vi "Main FPGA 8-axis with Limits.vi"() -> ()   [LabVIEW 2013]
uses:
  <vilib>/Motion/MotorControl/_s/nism.interpretControlRegister.stateTransition.ctl
  <vilib>/Platform/TimedLoop/XDataNode/timing_clust.ctl
  <vilib>/Platform/TimedLoop/XDataNode/nitl_modes.ctl
  <vilib>/Platform/TimedLoop/XDataNode/wakeup.ctl
  <vilib>/Motion/MotorControl/_s/nism.digitalInputs.portA.ctl
  <vilib>/rvi/Emulation/niFpgaSctlEmulationGetInTimedLoop.vi
  <vilib>/rvi/Emulation/niFpgaEmulationReportErrorSimple.vi
  <vilib>/rvi/Emulation/niFpgaGetClockAttributes.vi
  <vilib>/rvi/Emulation/niFpgaCriticalErrorInLSC.vi
  Global FPGA.vi
  <vilib>/rvi/eio/common/nirviEmuTemplateMethod_errors.vi
  <vilib>/Motion/SoftMotion/Synchronization/nism.rioScan.generateSyncScan.vi
  <vilib>/rvi/Emulation/niFpgaProcessEmulError.vi
  <vilib>/Motion/MotorControl/_s/nism.interpretControlRegister.indexed.vi
  <vilib>/Motion/MotorControl/_s/nism.generateStatusRegister.indexed.vi
  <vilib>/Motion/MotorControl/_s/nism.mdo.read.positionLoopSyncData.vi
  <vilib>/Motion/MotorControl/_s/nism.mdo.read.splineData.vi
  <vilib>/Motion/MotorControl/_s/nism.splineInterpolation.fxp.3.index.vi
  <vilib>/Motion/MotorControl/_s/nism.mdo.handler.indexed.vi
  <vilib>/Motion/MotorControl/_s/nism.digitalFilter.u8.vi
  <vilib>/Motion/MotorControl/_s/nism.interpretDIOControl.portA.single.2.vi
  <vilib>/Motion/MotorControl/_s/nism.generateDIOStatus.portA.single.vi
  <vilib>/Platform/TimedLoop/XDataNode/XDataNode.xnode
  <vilib>/eio/EIONode/EIONode.xnode
  <vilib>/Motion/MotorControl/NI_SoftMotion_MotorControlIP.lvlib
  <vilib>/Platform/TimedLoop/XDataNode/XDNodeRunTimeDep.lvlib
  <vilib>/Motion/SoftMotion/Synchronization/NI_SoftMotion_Synchronization.lvlib
panel:
  in  "Axis Digital Inputs (U8)":u8[](array[numeric])=[0, 0, 0, 0, 0, 0, 0, 0]
  out "Axis Positions":fxp<+/-,64,32>[](array[numeric])
  in  "STEP or CW? (T=STEP)":bool
  out "Drive Enable":bool[](array[boolean])
  in  "Enable Watchdog":bool
  in  "Pet Watchdog":bool
  in  "Watchdog Timeout Period (ticks)":u64=40000000 format="%.0p"
  out "Watchdog Timed Out?":bool
  out "Time Since Last Pet":u64
  in  "Enable value":bool
  in  "Drive Enable override?":bool
  out "State":T1=enum."Start --> Initializing" caption="state transition"
  in  "Sync Value":bool
  in  "Sync Enable override?":bool
  in  "Invert direction?":bool
  out "Sync is Fault":bool
  out "Sync is Locked":bool
  in  "minimum pulse":u16=40
  # "Synchronization Loop"
  # "Control Status Loop"
  # "Notes: \n1. This VI provides the communication interface between the NI SoftMotion Engine and the LabVIEW FPGA Module. You must compile this VI for a specific FPGA target before use. After compiling, run the VI before running any of the Express VI examples. For information on moving this example to another FPGA target, refer to ni.com/info and enter info code fpgaex.\n\n2. Only use the Reset Axis button if you are unable to communicate with the axis by any other means. This button resets the device state machine and other VIs to a known state. After resetting the axis, switch the NI Scan Engine from Active Mode to Configuration Mode, then back to Active Mode, before attempting to enable the axis."
  # "(These two buttons \nare for testing\npurposes.)"
  # "(These two buttons \nare for testing\npurposes.)"
  # "Step/Direction Loop"
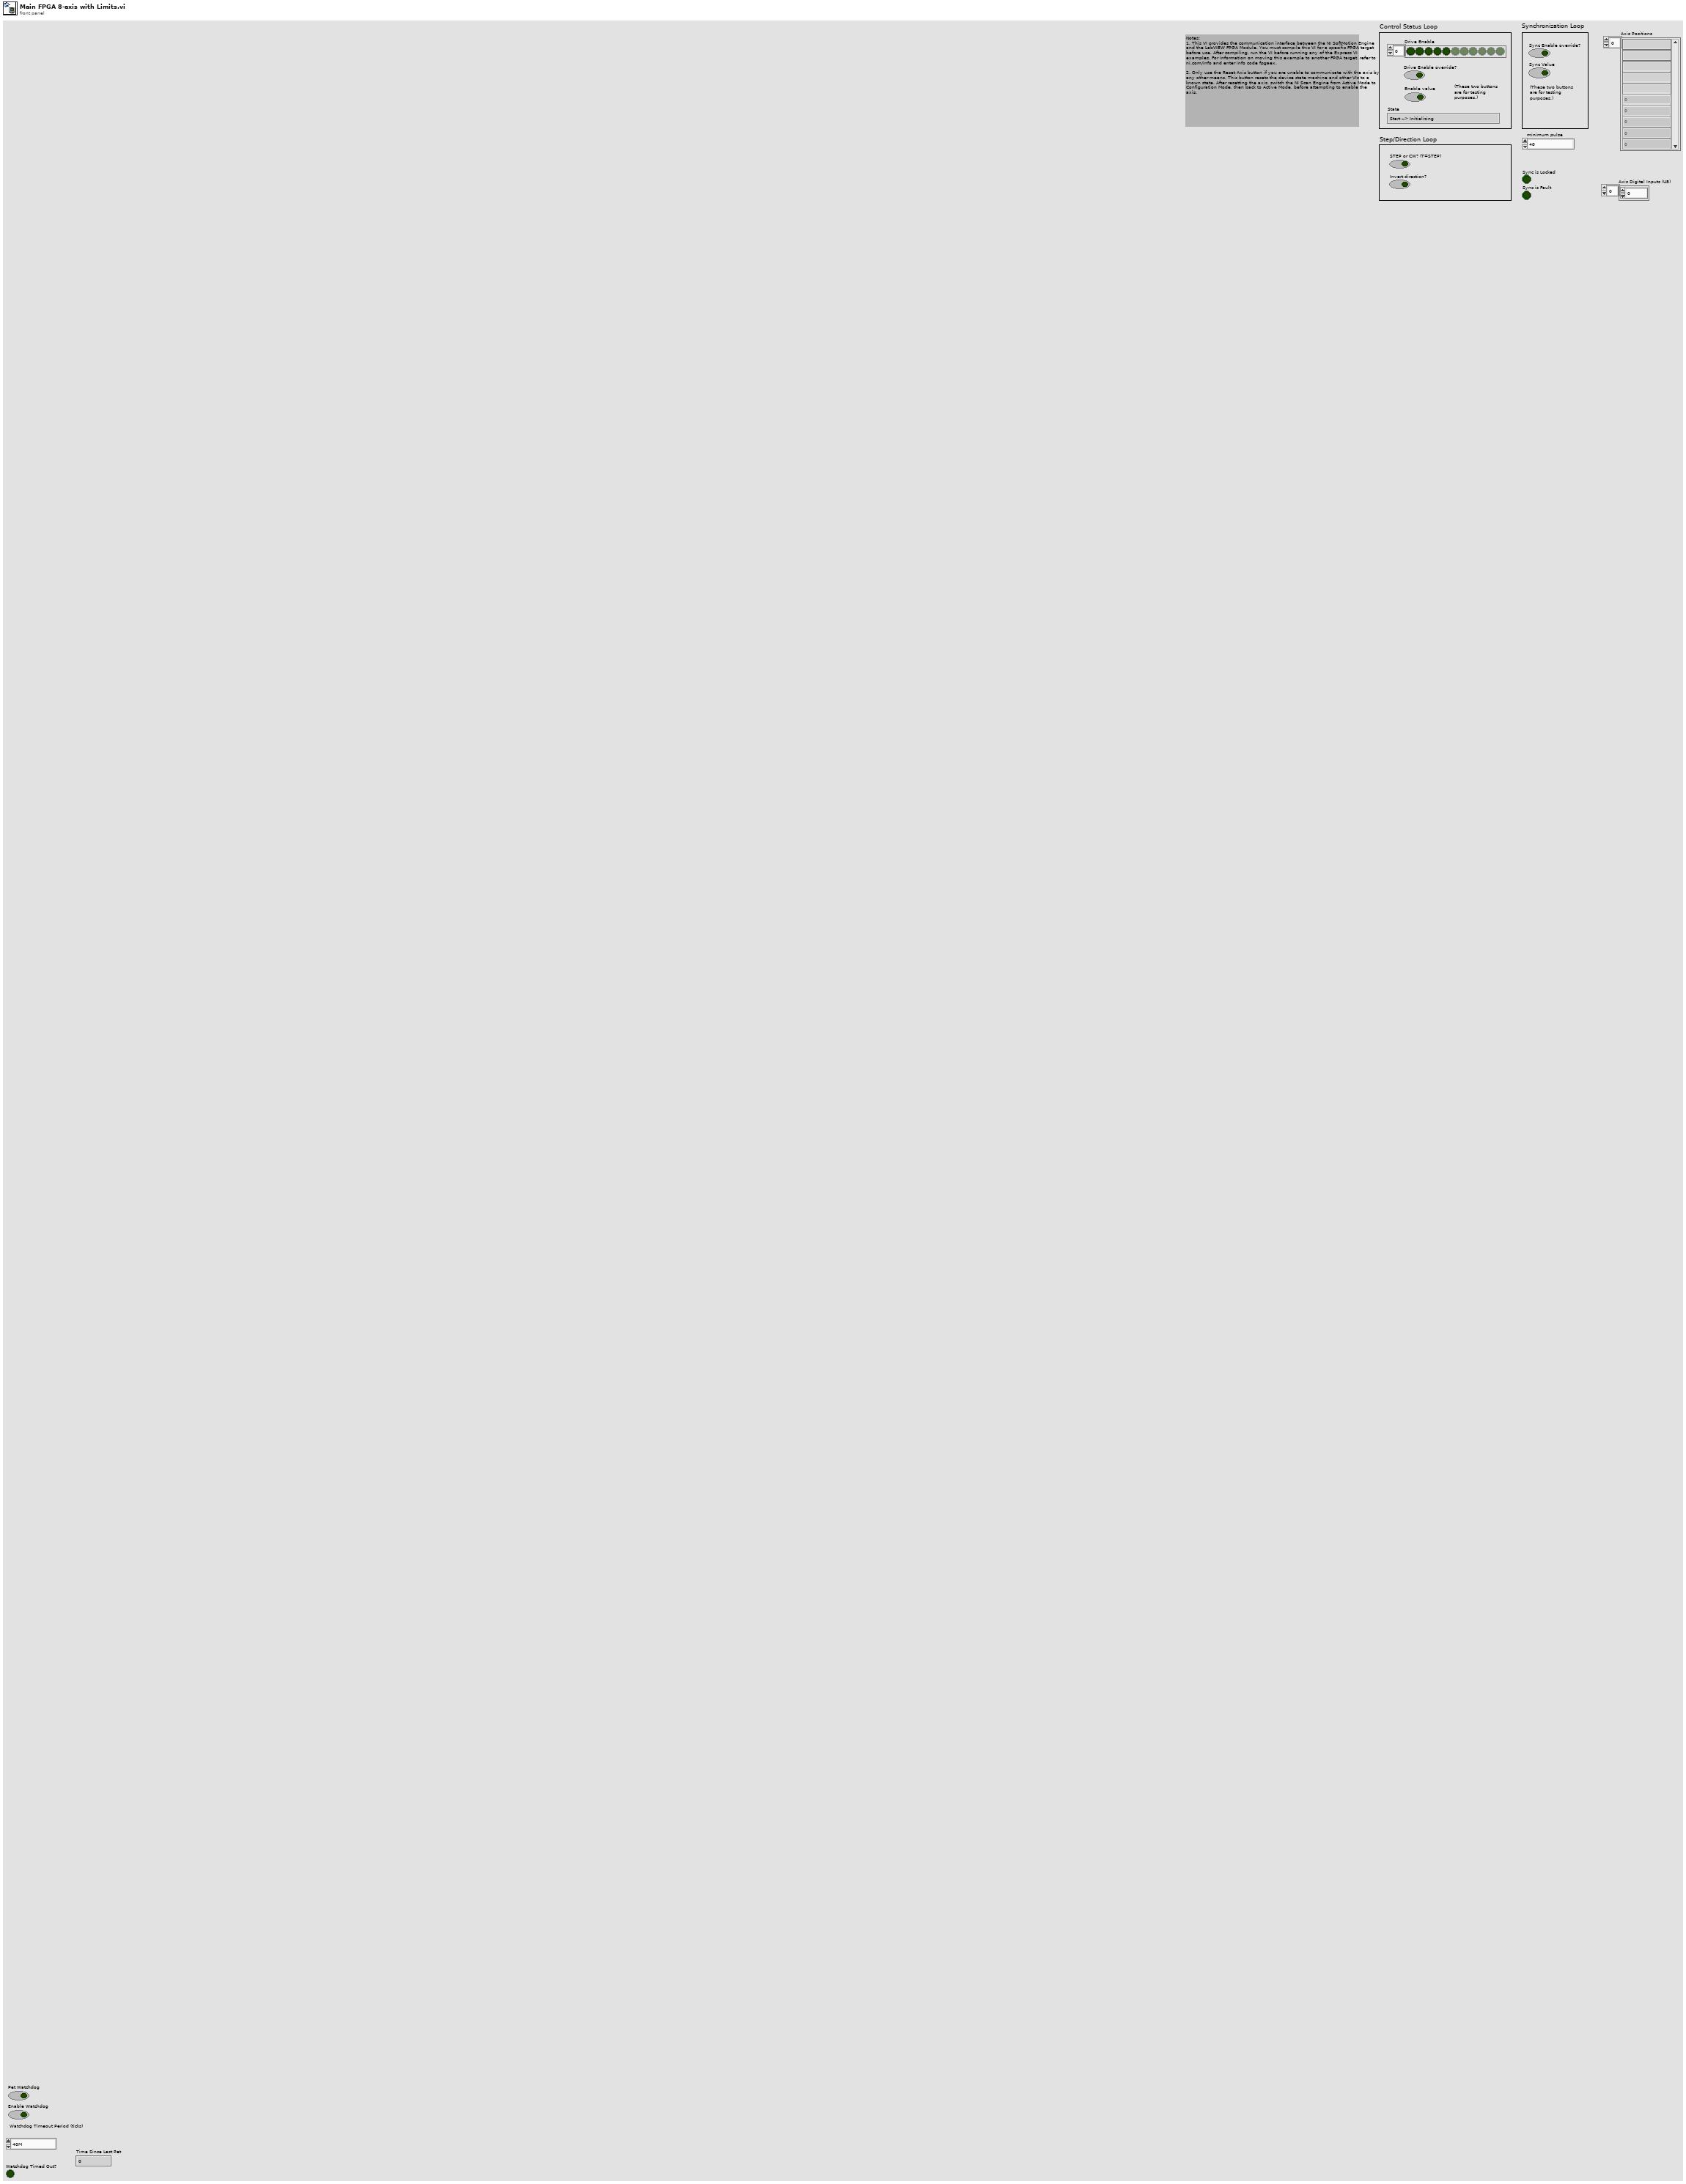
[diagram p1: front panel]
types:
  T1 = typedef "NI_SoftMotion_MotorControlIP.lvlib/nism.interpretControlRegister.stateTransition.ctl" = enum8{"Invalid", "Start --> Initializing", "Initializing --> Disabled", "Disabled --> Ready To Switch On", "Ready To Switch On --> Switched On", "Ready To Switch On --> Disable", "Switched On --> Operation Enable", "Switched On --> Ready To Switch On", "Switched On --> Disabled", "Operation Enable --> Switched On", "Operation Enable --> Ready To Switch On", "Operation Enable --> Disabled", "Fault --> Disabled", "Any --> Fault", "None"}
  T2 = typedef "NI_SoftMotion_MotorControlIP.lvlib/nism.mdo.splineData.ctl" = cluster{"spline type":T3, "traj per/spline per":u16, "spline per/traj per":fxp<+,32,0>}
  T3 = typedef "nism.splineInterpolation.type.ctl" = u16
  T4 = typedef "NI_SoftMotion_Synchronization.lvlib/nism.softmotionScan.timerConfig.ctl" = cluster{"Target Period (clocks)":u16, "Host Period / Target Period":u16}
  T5 = typedef "NI_SoftMotion_Synchronization.lvlib/nism.softmotionScan.timerControl.ctl" = cluster{"SM Scan":bool, "SM Scan Count":u32, "SM Scan Enabled":bool}
  T6 = typedef "XDNodeRunTimeDep.lvlib/timing_clust.ctl" = cluster{"Expected End [f-1]":u64, "Actual End [f-1]":u64, "Finished Late? [f-1]":bool, "Expected End [i-1]":u64, "Actual End [i-1]":u64, "Finished Late? [i-1]":bool, "Expected Start [i]":u64, "Actual Start [i]":u64, "Expected Start [f]":u64, "Actual Start [f]":u64, "Source Name":string, "Structure Name":string, "Period":i64, "Deadline":i64, "Offset":i64, "Start":i64, "Priority":i32, "Timeout":i32, "Mode":T7, "Wakeup Reason":T8, "Error":errorcluster, "Source Type":string, "Secondary Source Type":string, "Global End Time":u64, "Global Start Time":u64, "Frame Duration":u64, "Iteration Duration":u64, "Assigned CPU":i32, "I/O Scan Engine Mode":u32}
  T7 = typedef "XDNodeRunTimeDep.lvlib/nitl_modes.ctl" = enum32{"No Change", "Process missed periods, maintain original phase", "Discard missed periods, maintain original phase", "Process missed periods, ignore original phase", "Discard missed periods, ignore original phase"}
  T8 = typedef "XDNodeRunTimeDep.lvlib/wakeup.ctl" = enum32{"Normal", "Aborted", "Asynchronous wakeup", "Timing source error", "Timed loop error", "Timeout"}
  T9 = typedef "NI_SoftMotion_MotorControlIP.lvlib/nism.digitalInputs.portA.ctl" = cluster{"reverse limit":bool, "forward limit":bool, "home switch":bool, "digital input 0":bool, "digital input 1":bool, "digital input 2":bool, "digital input 3":bool}
  T10 = typedef "NI_SoftMotion_MotorControlIP.lvlib/nism.dio.portA.config.2.ctl" = cluster{"digital filter (us)":u16[], "safe state":enum16{"Low", "High", "No Change"}[]}
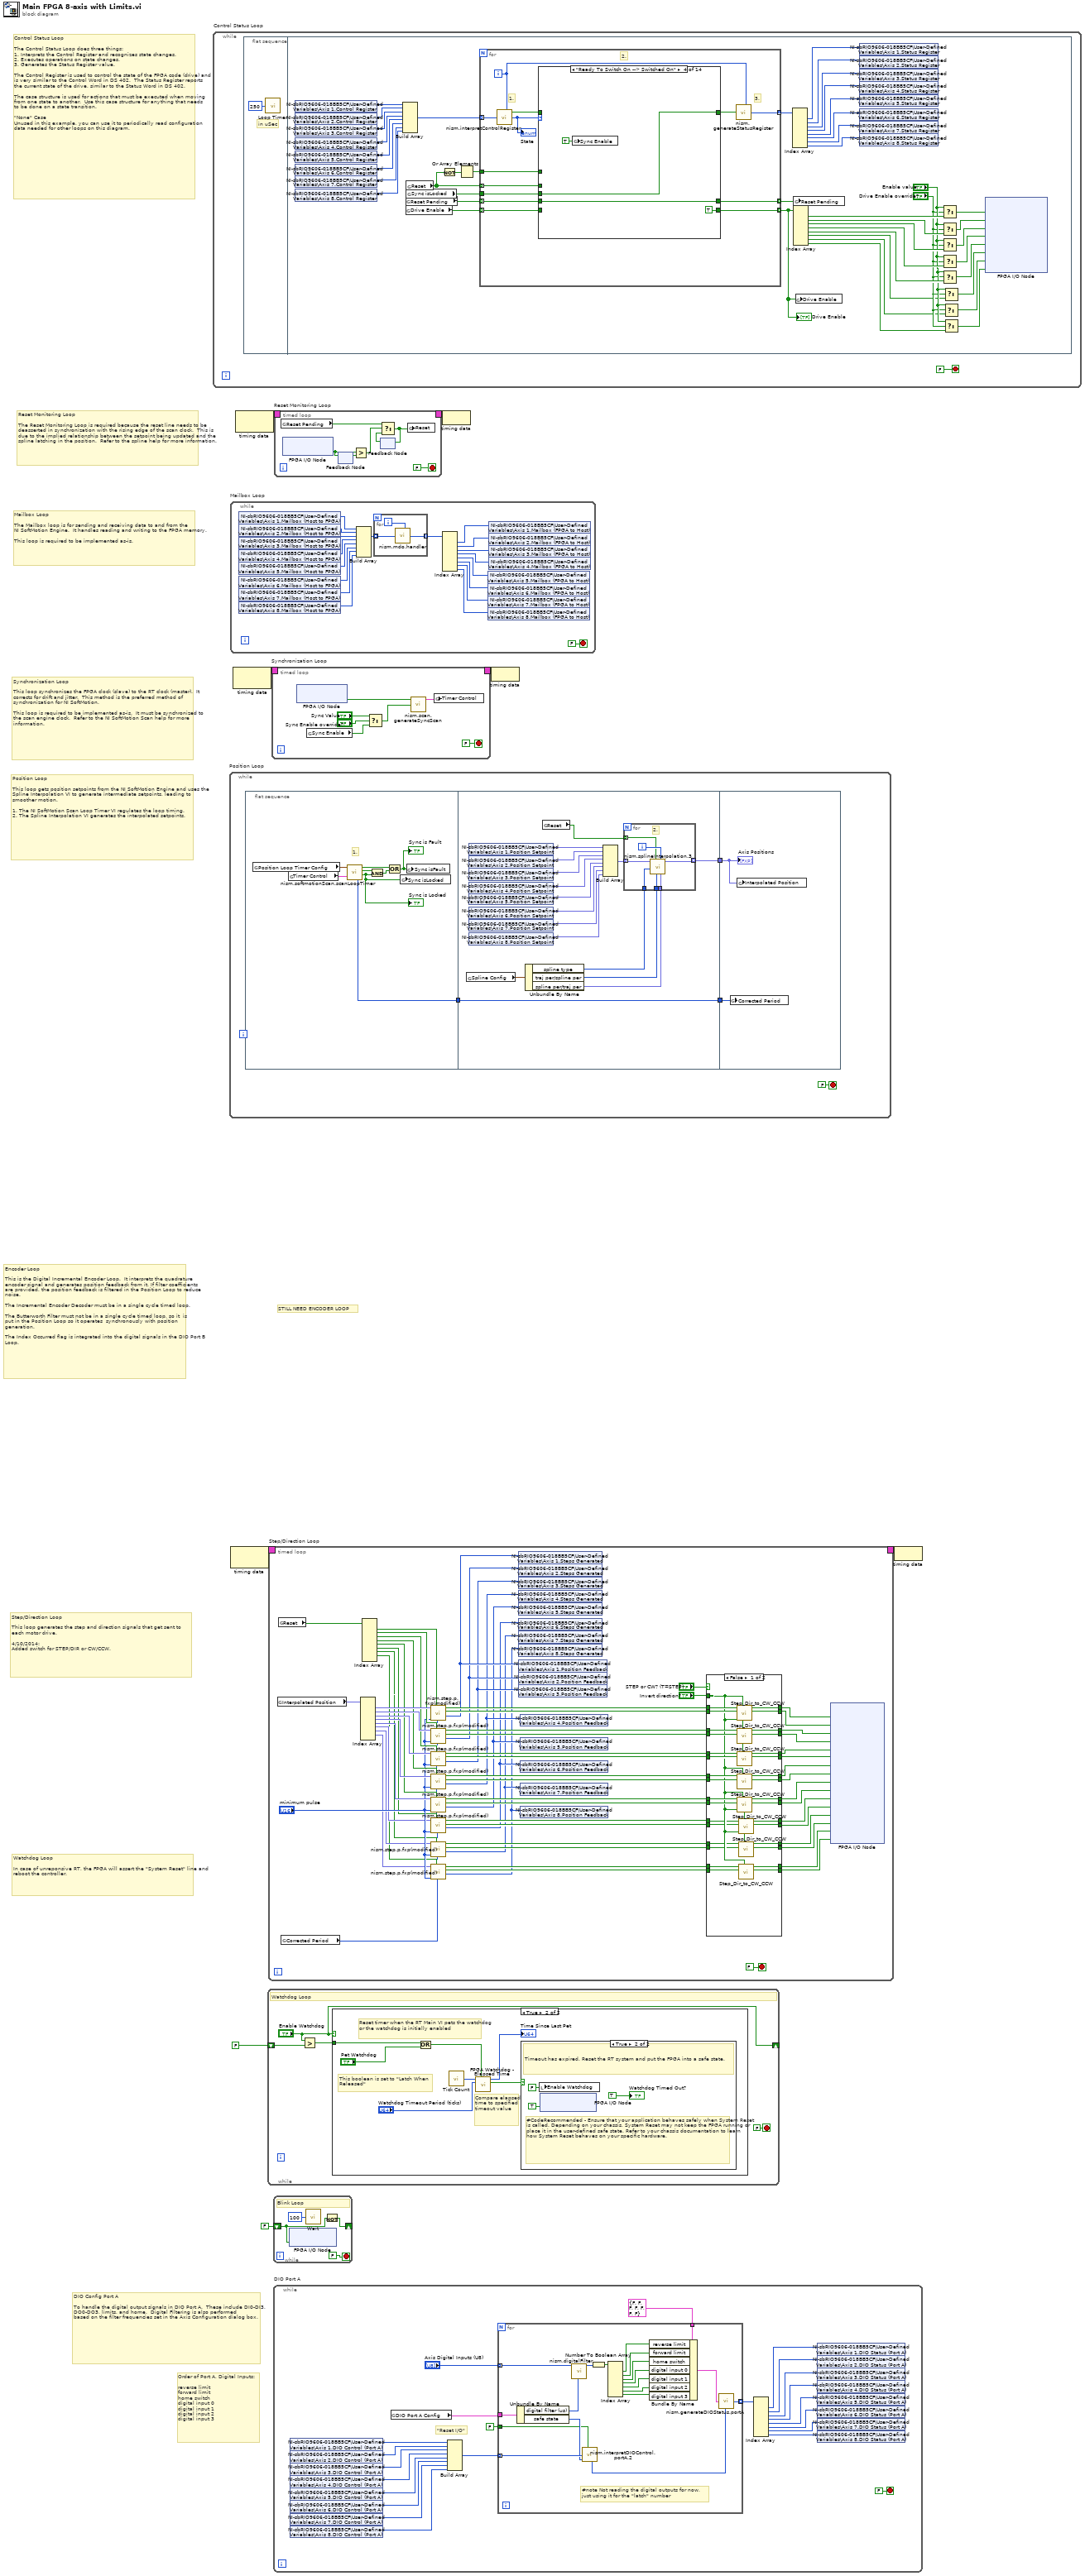
[diagram p0: block diagram]
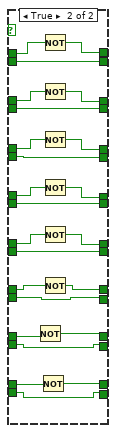
[diagram p5: hidden frame]
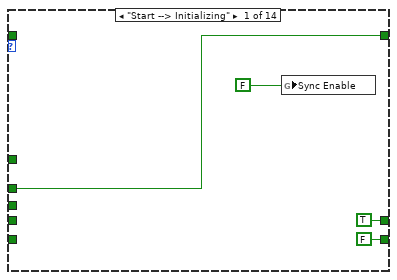
[diagram p6: hidden frame]
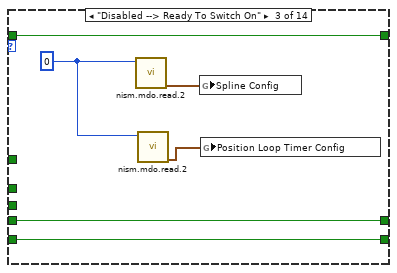
[diagram p8: hidden frame]
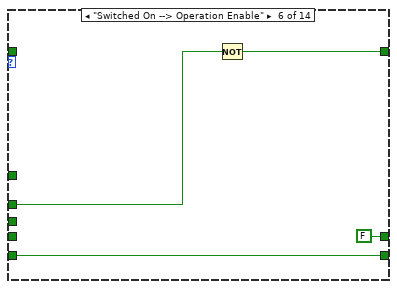
[diagram p10: hidden frame]
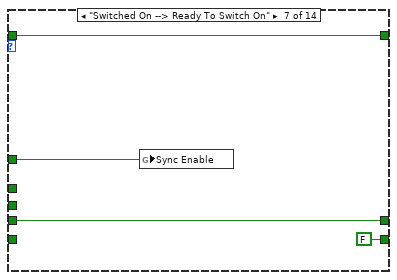
[diagram p11: hidden frame]
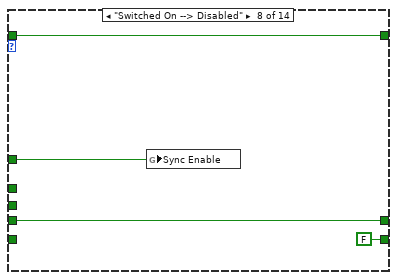
[diagram p12: hidden frame]
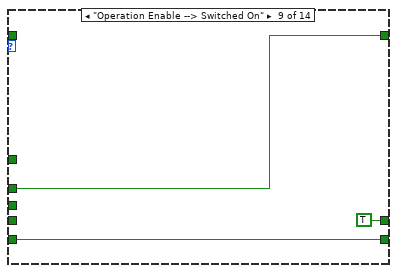
[diagram p13: hidden frame]
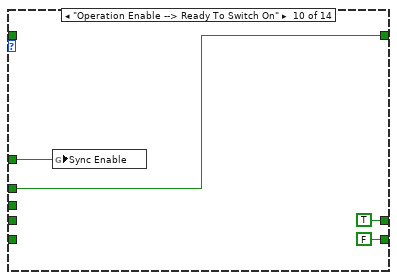
[diagram p14: hidden frame]
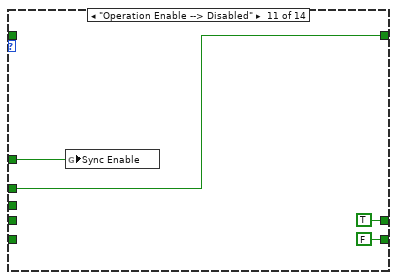
[diagram p15: hidden frame]
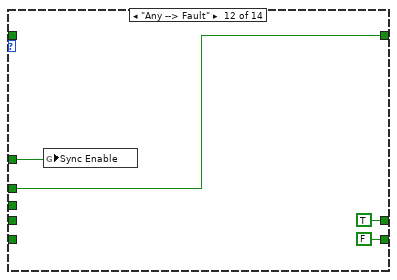
[diagram p16: hidden frame]
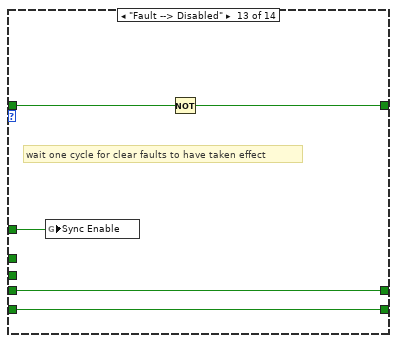
[diagram p17: hidden frame]
diagram:
  # "STILL NEED ENCODER LOOP"
  # "DIO Config Port A\n\nTo handle the digital output signals in DIO Port A.  These include DI0-DI3, DO0-DO3, limits, and home.  Digital Filtering is also performed\nbased on the filter frequencies set in the Axis Configuration dialog box."
  # "Order of Port A, Digital Inputs:\n\nreverse limit\nforward limit\nhome switch\ndigital input 0\ndigital input 1\ndigital input 2\ndigital input 3"
  # "Encoder Loop\n\nThis is the Digital Incremental Encoder Loop.  It interprets the quadrature encoder signal and generates position feedback from it. If filter coefficients are provided, the position feedback is filtered in the Position Loop to reduce noise.\n\nThe Incremental Encoder Decoder must be in a single cycle timed loop.\n\nThe Butterworth Filter must not be in a single cycle timed loop, so it  is\nput in the Position Loop so it operates  synchronously with position generation.\n\nThe Index Occurred flag is integrated into the digital signals in the DIO Port B Loop."
  # "Watchdog Loop\n\nIn case of unreponsive RT, the FPGA will assert the \"System Reset\" line and reboot the controller."
  # "Step/Direction Loop\n\nThis loop generates the step and direction signals that get sent to \neach motor drive.\n\n4/10/2014:\nAdded switch for STEP/DIR or CW/CCW."
  # "Position Loop\n\nThis loop gets position setpoints from the NI SoftMotion Engine and uses the Spline Interpolation VI to generate intermediate setpoints, leading to smoother motion.\n\n1. The NI SoftMotion Scan Loop Timer VI regulates the loop timing. \n2. The Spline Interpolation VI generates the interpolated setpoints."
  # "Synchronization Loop\n\nThis loop synchronizes the FPGA clock (slave) to the RT clock (master).  It corrects for drift and jitter.  This method is the preferred method of synchronization for NI SoftMotion.\n\nThis loop is required to be implemented as-is.  It must be synchronized to the scan engine clock.  Refer to the NI SoftMotion Scan help for more information."
  # "Mailbox Loop\n\nThe Mailbox loop is for sending and receiving data to and from the \nNI SoftMotion Engine.  It handles reading and writing to the FPGA memory.\n\nThis loop is required to be implemented as-is."
  # "Reset Monitoring Loop\n\nThe Reset Monitoring Loop is required because the reset line needs to be deasserted in synchronization with the rising edge of the scan clock.  This is due to the implied relationship between the setpoint being updated and the spline latching in the position.  Refer to the spline help for more information."
  # "Control Status Loop\n\nThe Control Status Loop does three things:\n1. Interprets the Control Register and recognizes state changes.\n2. Executes operations on state changes.\n3. Generates the Status Register value.\n\nThe Control Register is used to control the state of the FPGA code (drive) and is very similar to the Control Word in DS 402.  The Status Register reports the current state of the drive, similar to the Status Word in DS 402.\n\nThe case structure is used for actions that must be executed when moving from one state to another.  Use this case structure for anything that needs to be done on a state transition.\n\n\"None\" Case\nUnused in this example, you can use it to periodically read configuration data needed for other loops on this diagram."
  n1 = while "Control Status Loop" {
    stop <- FALSE stop-if-true
    n2 = flat-sequence {
      frame #0 {
        # "in uSec"
        n3 = call "Loop Timer"("Count(uSec)"=u32 250) -> ()  [unwired: 1 out]
      }
      frame #1 {
        n4 = shared-variable "NI-sbRIO9606-018BB5CF\\User-Defined Variables\\Axis 1.Control Register"() -> (w44:u32)  [unwired: 1 in, 1 out]
        n5 = shared-variable "NI-sbRIO9606-018BB5CF\\User-Defined Variables\\Axis 2.Control Register"() -> (w43:u32)  [unwired: 1 in, 1 out]
        n6 = shared-variable "NI-sbRIO9606-018BB5CF\\User-Defined Variables\\Axis 3.Control Register"() -> (w42:u32)  [unwired: 1 in, 1 out]
        n7 = shared-variable "NI-sbRIO9606-018BB5CF\\User-Defined Variables\\Axis 4.Control Register"() -> (w41:u32)  [unwired: 1 in, 1 out]
        n8 = shared-variable "NI-sbRIO9606-018BB5CF\\User-Defined Variables\\Axis 5.Control Register"() -> (w40:u32)  [unwired: 1 in, 1 out]
        n9 = shared-variable "NI-sbRIO9606-018BB5CF\\User-Defined Variables\\Axis 6.Control Register"() -> (w24:u32)  [unwired: 1 in, 1 out]
        n10 = shared-variable "NI-sbRIO9606-018BB5CF\\User-Defined Variables\\Axis 7.Control Register"() -> (w23:u32)  [unwired: 1 in, 1 out]
        n11 = shared-variable "NI-sbRIO9606-018BB5CF\\User-Defined Variables\\Axis 8.Control Register"() -> (w22:u32)  [unwired: 1 in, 1 out]
        n12 = Build Array(w44, w43, w42, w41, w40, w24, w23, w22) -> (w53:u32[])
        n13 = global read "Global FPGA.vi" "Reset Pending"() -> (w48:bool[])
        n14 = global read "Global FPGA.vi" "Drive Enable"() -> (w47:bool[])
        n15 = global read "Global FPGA.vi" "Reset"() -> (w49:bool[])
        n16 = global read "Global FPGA.vi" "Sync isLocked"() -> (w54:bool)
        n17 = Not(x=w49) -> (.not. x?=w51:bool[])
        n18 = Or Array Elements(Boolean array=w51) -> (logical OR=w50:bool)
        n19 = for {
          tunnel: w49 -> [w62] mode=indexing
          tunnel: w54 -> [w61]
          tunnel: w53 -> [w63] mode=indexing
          tunnel: [w60] -> w45 mode=indexing
          tunnel: [w59] -> w52 mode=indexing
          tunnel: [w58] -> w46 mode=indexing
          tunnel: w50 -> [w57]
          tunnel: w48 -> [w56] mode=indexing
          tunnel: w47 -> [w55] mode=indexing
          i -> [w64]
          # "3."
          # "2."
          # "1."
          n20 = call-poly <vilib>:"nism.interpretControlRegister.vi"("control register"=w63, "axis index"=w64) -> ("transition occurred"=w65:bool, "state transition"=w66:T1)  [unwired: 6 in]
          "State" <- w66
          n21 = case shown="\"Ready To Switch On --> Switched On\"" w66 {
            tunnel: w65 -> [_ w74 w80 _ w87 _ w95 w99 _ _ _ _ w119 _]
            tunnel: [w71 w74 w80 w82 w87 w91 w95 w99 w101 w104 w108 w112 w118 _] -> w67
            tunnel: w62 -> [w71 _ _ _ _ w90 _ _ w101 w104 w108 w112 _ _]
            tunnel: w61 -> [_ _ _ w82 _ _ _ _ _ _ _ _ _ _]
            tunnel: [TRUE ("Write.Reset Pending") w73 w76 w81 w86 FALSE ("Write.Reset Pending") w92 w96 TRUE ("Write.Reset Pending") TRUE ("Write.Reset Pending") TRUE ("Write.Reset Pending") TRUE ("Write.Reset Pending") w116 w121] -> w59
            tunnel: [FALSE ("Write.Drive Enable") w72 w75 TRUE ("Write.Drive Enable") w85 w88 FALSE ("Write.Drive Enable") FALSE ("Write.Drive Enable") w100 FALSE ("Write.Drive Enable") FALSE ("Write.Drive Enable") FALSE ("Write.Drive Enable") w115 w120] -> w58
            tunnel: w57 -> [_ _ _ _ _ _ w93 w97 _ w103 w107 w111 w117 _]
            tunnel: w56 -> [_ w73 w76 w81 w86 _ w92 w96 _ _ _ _ w116 w121]
            tunnel: w55 -> [_ w72 w75 _ w85 w88 _ _ w100 _ _ _ w115 w120]
            frame "Start --> Initializing" {
              n22 = global write "Global FPGA.vi" "Sync Enable"(FALSE ("Sync Enable")) -> ()
            }
            frame "Initializing --> Disabled" {
            }
            frame "Disabled --> Ready To Switch On" {
              w78 = 0 ("axis index")
              n23 = call-poly <vilib>:"nism.mdo.read.2.vi"("axis index"=w78) -> ("spline"=w79:T2)  [unwired: 10 in]
              n24 = call-poly <vilib>:"nism.mdo.read.2.vi"("axis index"=w78) -> ("position loop sync"=w77:T4)  [unwired: 10 in]
              n25 = global write "Global FPGA.vi" "Spline Config"(w79) -> ()
              n26 = global write "Global FPGA.vi" "Position Loop Timer Config"(w77) -> ()
            }
            frame "Ready To Switch On --> Switched On" {
              n27 = global write "Global FPGA.vi" "Sync Enable"(TRUE ("Sync Enable")) -> ()
            }
            frame "Ready To Switch On --> Disable" {
            }
            frame "Switched On --> Operation Enable" {
              n28 = Not(x=w90) -> (.not. x?=w91:bool)
            }
            frame "Switched On --> Ready To Switch On" {
              n29 = global write "Global FPGA.vi" "Sync Enable"(w93) -> ()
            }
            frame "Switched On --> Disabled" {
              n30 = global write "Global FPGA.vi" "Sync Enable"(w97) -> ()
            }
            frame "Operation Enable --> Switched On" {
            }
            frame "Operation Enable --> Ready To Switch On" {
              n31 = global write "Global FPGA.vi" "Sync Enable"(w103) -> ()
            }
            frame "Operation Enable --> Disabled" {
              n32 = global write "Global FPGA.vi" "Sync Enable"(w107) -> ()
            }
            frame "Any --> Fault" {
              n33 = global write "Global FPGA.vi" "Sync Enable"(w111) -> ()
            }
            frame "Fault --> Disabled" {
              # "wait one cycle for clear faults to have taken effect"
              n34 = global write "Global FPGA.vi" "Sync Enable"(w117) -> ()
              n35 = Not(x=w119) -> (.not. x?=w118:bool)
            }
            frame "None", Default {
            }
          }
          n36 = call-poly <vilib>:"nism.generateStatusRegister.vi"("transition success"=w67, "axis index"=w64) -> ("status register"=w60:u32)  [unwired: 7 in]
        }
        "Drive Enable" <- w46
        n37 = Index Array(array=w45) -> (element #1=w39:u32, element #2=w38:u32, element #3=w37:u32, element #4=w36:u32, element #5=w35:u32, element #6=w21:u32, element #7=w20:u32, element #8=w19:u32)  [unwired: 8 in]
        n38 = global write "Global FPGA.vi" "Reset Pending"(w52) -> ()
        n39 = Index Array(array=w46) -> (element #1=w34:bool, element #2=w32:bool, element #3=w30:bool, element #4=w28:bool, element #5=w26:bool, element #6=w16:bool, element #7=w15:bool, element #8=w14:bool)  [unwired: 8 in]
        n40 = global write "Global FPGA.vi" "Drive Enable"(w46) -> ()
        n41 = shared-variable "NI-sbRIO9606-018BB5CF\\User-Defined Variables\\Axis 1.Status Register"(w39) -> ()  [unwired: 1 in, 1 out]
        n42 = shared-variable "NI-sbRIO9606-018BB5CF\\User-Defined Variables\\Axis 2.Status Register"(w38) -> ()  [unwired: 1 in, 1 out]
        n43 = shared-variable "NI-sbRIO9606-018BB5CF\\User-Defined Variables\\Axis 3.Status Register"(w37) -> ()  [unwired: 1 in, 1 out]
        n44 = shared-variable "NI-sbRIO9606-018BB5CF\\User-Defined Variables\\Axis 4.Status Register"(w36) -> ()  [unwired: 1 in, 1 out]
        n45 = shared-variable "NI-sbRIO9606-018BB5CF\\User-Defined Variables\\Axis 5.Status Register"(w35) -> ()  [unwired: 1 in, 1 out]
        n46 = shared-variable "NI-sbRIO9606-018BB5CF\\User-Defined Variables\\Axis 6.Status Register"(w21) -> ()  [unwired: 1 in, 1 out]
        n47 = shared-variable "NI-sbRIO9606-018BB5CF\\User-Defined Variables\\Axis 7.Status Register"(w20) -> ()  [unwired: 1 in, 1 out]
        n48 = shared-variable "NI-sbRIO9606-018BB5CF\\User-Defined Variables\\Axis 8.Status Register"(w19) -> ()  [unwired: 1 in, 1 out]
        n49 = Select(t="Enable value", s="Drive Enable override?", f=w34) -> (s? t:f=w33:bool)
        n50 = Select(t="Enable value", s="Drive Enable override?", f=w32) -> (s? t:f=w31:bool)
        n51 = Select(t="Enable value", s="Drive Enable override?", f=w30) -> (s? t:f=w29:bool)
        n52 = Select(t="Enable value", s="Drive Enable override?", f=w28) -> (s? t:f=w27:bool)
        n53 = Select(t="Enable value", s="Drive Enable override?", f=w26) -> (s? t:f=w25:bool)
        n54 = Select(t="Enable value", s="Drive Enable override?", f=w16) -> (s? t:f=w13:bool)
        n55 = Select(t="Enable value", s="Drive Enable override?", f=w15) -> (s? t:f=w12:bool)
        n56 = Select(t="Enable value", s="Drive Enable override?", f=w14) -> (s? t:f=w11:bool)
        n57 = xnode "FPGA I/O Node"("Axis1_Servo On"=w33, "Axis2_Servo On"=w31, "Axis3_Servo On"=w29, "Axis4_Servo On"=w27, "Axis5_Servo On"=w25, "RMC/DIO1"=w13, "RMC/DIO2"=w12, "RMC/DIO3"=w11) -> ()  [unwired: 8 in, 8 out]
      }
    }
  }
  n58 = while "Position Loop" {
    stop <- FALSE stop-if-true
    n59 = flat-sequence {
      tunnel: [w126] -> w122
      tunnel: [w143] -> w124
      tunnel: [w142] -> w123
      tunnel: w122 -> [w142]
      tunnel: w124 -> [w157]
      tunnel: w123 -> [w158]
      frame #0 {
        # "1."
        n60 = global read "Global FPGA.vi" "Position Loop Timer Config"() -> (w128:T4)
        n61 = global read "Global FPGA.vi" "Timer Control"() -> (w127:T5)
        n62 = call <vilib>:"nism.softmotionScan.scanLoopTimer.vi"("Timer Control"=w127, "Timer Config"=w128) -> ("Scan Running?"=w130:bool, "Finished Late?"=w132:bool, "Fault Occurred?"=w133:bool, "Corrected Period"=w126:u16)  [unwired: 5 in, 1 out]
        "Sync is Locked" <- w130
        n63 = Compound Arithmetic op=AND(w132, w130) -> (w131:bool)
        n64 = Compound Arithmetic op=OR(w133, w131) -> (w129:bool)
        "Sync is Fault" <- w129
        n65 = global write "Global FPGA.vi" "Sync isLocked"(w130) -> ()
        n66 = global write "Global FPGA.vi" "Sync isFault"(w129) -> ()
      }
      frame #1 {
        n67 = global read "Global FPGA.vi" "Spline Config"() -> (w145:T2)
        n68 = shared-variable "NI-sbRIO9606-018BB5CF\\User-Defined Variables\\Axis 1.Position Setpoint"() -> (w141:fxp<+/-,64,32>)  [unwired: 1 in, 1 out]
        n69 = shared-variable "NI-sbRIO9606-018BB5CF\\User-Defined Variables\\Axis 2.Position Setpoint"() -> (w140:fxp<+/-,64,32>)  [unwired: 1 in, 1 out]
        n70 = shared-variable "NI-sbRIO9606-018BB5CF\\User-Defined Variables\\Axis 3.Position Setpoint"() -> (w139:fxp<+/-,64,32>)  [unwired: 1 in, 1 out]
        n71 = shared-variable "NI-sbRIO9606-018BB5CF\\User-Defined Variables\\Axis 4.Position Setpoint"() -> (w138:fxp<+/-,64,32>)  [unwired: 1 in, 1 out]
        n72 = shared-variable "NI-sbRIO9606-018BB5CF\\User-Defined Variables\\Axis 5.Position Setpoint"() -> (w137:fxp<+/-,64,32>)  [unwired: 1 in, 1 out]
        n73 = shared-variable "NI-sbRIO9606-018BB5CF\\User-Defined Variables\\Axis 6.Position Setpoint"() -> (w136:fxp<+/-,64,32>)  [unwired: 1 in, 1 out]
        n74 = shared-variable "NI-sbRIO9606-018BB5CF\\User-Defined Variables\\Axis 7.Position Setpoint"() -> (w135:fxp<+/-,64,32>)  [unwired: 1 in, 1 out]
        n75 = shared-variable "NI-sbRIO9606-018BB5CF\\User-Defined Variables\\Axis 8.Position Setpoint"() -> (w134:fxp<+/-,64,32>)  [unwired: 1 in, 1 out]
        n76 = Unbundle By Name(w145) -> ("spline type"=w149:T3, "traj per/spline per"=w148:u16, "spline per/traj per"=w147:fxp<+,32,0>)
        n77 = global read "Global FPGA.vi" "Reset"() -> (w144:bool[])
        n78 = Build Array(w141, w140, w139, w138, w137, w136, w135, w134) -> (w146:fxp<+/-,64,32>[])
        n79 = for {
          tunnel: w149 -> [w156]
          tunnel: w148 -> [w155]
          tunnel: w147 -> [w154]
          tunnel: w144 -> [w151] mode=indexing
          tunnel: w146 -> [w153] mode=indexing
          tunnel: [w150] -> w143 mode=indexing
          i -> [w152]
          # "2."
          n80 = call-poly <vilib>:"nism.splineInterpolation.3.vi"("1 / calls per sample"=w154, "index"=w152, "calls per sample"=w155, "reset"=w151, "spline type"=w156, "x"=w153) -> ("xi"=w150:fxp<+/-,64,32>)  [unwired: 5 in]
        }
      }
      frame #2 {
        n81 = global write "Global FPGA.vi" "Corrected Period"(w158) -> ()
        n82 = global write "Global FPGA.vi" "Interpolated Position"(w157) -> ()
        "Axis Positions" <- w157
      }
    }
  }
  n83 = while "Mailbox Loop" {
    stop <- FALSE stop-if-true
    n84 = shared-variable "NI-sbRIO9606-018BB5CF\\User-Defined Variables\\Axis 1.Mailbox (Host to FPGA)"() -> (w174:u64)  [unwired: 1 in, 1 out]
    n85 = shared-variable "NI-sbRIO9606-018BB5CF\\User-Defined Variables\\Axis 2.Mailbox (Host to FPGA)"() -> (w173:u64)  [unwired: 1 in, 1 out]
    n86 = shared-variable "NI-sbRIO9606-018BB5CF\\User-Defined Variables\\Axis 3.Mailbox (Host to FPGA)"() -> (w172:u64)  [unwired: 1 in, 1 out]
    n87 = shared-variable "NI-sbRIO9606-018BB5CF\\User-Defined Variables\\Axis 4.Mailbox (Host to FPGA)"() -> (w171:u64)  [unwired: 1 in, 1 out]
    n88 = shared-variable "NI-sbRIO9606-018BB5CF\\User-Defined Variables\\Axis 5.Mailbox (Host to FPGA)"() -> (w170:u64)  [unwired: 1 in, 1 out]
    n89 = shared-variable "NI-sbRIO9606-018BB5CF\\User-Defined Variables\\Axis 6.Mailbox (Host to FPGA)"() -> (w164:u64)  [unwired: 1 in, 1 out]
    n90 = shared-variable "NI-sbRIO9606-018BB5CF\\User-Defined Variables\\Axis 7.Mailbox (Host to FPGA)"() -> (w163:u64)  [unwired: 1 in, 1 out]
    n91 = shared-variable "NI-sbRIO9606-018BB5CF\\User-Defined Variables\\Axis 8.Mailbox (Host to FPGA)"() -> (w162:u64)  [unwired: 1 in, 1 out]
    n92 = Build Array(w174, w173, w172, w171, w170, w164, w163, w162) -> (w176:u64[])
    n93 = for {
      tunnel: w176 -> [w180] mode=indexing
      tunnel: [w179] -> w175 mode=indexing
      i -> [w178]
      n94 = call-poly <vilib>:"nism.mdo.handler.vi"("mbox (host to fpga)"=w180, "axis index"=w178) -> ("mbox (fpga to host)"=w179:u64)  [unwired: 7 in]
    }
    n95 = Index Array(array=w175) -> (element #1=w169:u64, element #2=w168:u64, element #3=w167:u64, element #4=w166:u64, element #5=w165:u64, element #6=w161:u64, element #7=w160:u64, element #8=w159:u64)  [unwired: 8 in]
    n96 = shared-variable "NI-sbRIO9606-018BB5CF\\User-Defined Variables\\Axis 6.Mailbox (FPGA to Host)"(w161) -> ()  [unwired: 1 in, 1 out]
    n97 = shared-variable "NI-sbRIO9606-018BB5CF\\User-Defined Variables\\Axis 7.Mailbox (FPGA to Host)"(w160) -> ()  [unwired: 1 in, 1 out]
    n98 = shared-variable "NI-sbRIO9606-018BB5CF\\User-Defined Variables\\Axis 8.Mailbox (FPGA to Host)"(w159) -> ()  [unwired: 1 in, 1 out]
    n99 = shared-variable "NI-sbRIO9606-018BB5CF\\User-Defined Variables\\Axis 5.Mailbox (FPGA to Host)"(w165) -> ()  [unwired: 1 in, 1 out]
    n100 = shared-variable "NI-sbRIO9606-018BB5CF\\User-Defined Variables\\Axis 1.Mailbox (FPGA to Host)"(w169) -> ()  [unwired: 1 in, 1 out]
    n101 = shared-variable "NI-sbRIO9606-018BB5CF\\User-Defined Variables\\Axis 2.Mailbox (FPGA to Host)"(w168) -> ()  [unwired: 1 in, 1 out]
    n102 = shared-variable "NI-sbRIO9606-018BB5CF\\User-Defined Variables\\Axis 3.Mailbox (FPGA to Host)"(w167) -> ()  [unwired: 1 in, 1 out]
    n103 = shared-variable "NI-sbRIO9606-018BB5CF\\User-Defined Variables\\Axis 4.Mailbox (FPGA to Host)"(w166) -> ()  [unwired: 1 in, 1 out]
  }
  n104 = node-c288() -> (w8:T6)  [unwired: 1 in]
  n105 = node-c288() -> (w6:T6)  [unwired: 1 in]
  n106 = node-c288() -> (w4:T6)  [unwired: 1 in]
  n107 = while "RT Watchdog Loop" {
    shift-right: ["Enable Watchdog"] -> _
    shift-left: FALSE ("Enable RT Watchdog") -> [w184]
    stop <- FALSE stop-if-true
    # "Watchdog Loop"
    n108 = Greater?(x="Enable Watchdog", y=w184) -> (0:w181:bool)
    n109 = case shown="True" "Enable Watchdog" {
      tunnel: w181 -> [_ w187]
      frame False {
        # "This loop has to be explicitly enabled from the RT Main VI.  This reduces the possiblity of an endless reboot cycle."
      }
      frame True {
        # "This boolean is set to \"Latch When Released\""
        # "Compare elapsed time to specified timeout value"
        # "Reset timer when the RT Main VI pets the watchdog or the watchdog is initially enabled"
        n110 = Or(x=w187, y="Pet Watchdog") -> (x .or. y?=w186:bool)
        n111 = call "Tick Count"() -> ("Tick Count(Ticks)"=w190:u32)
        n112 = call "FPGA Watchdog - Elapsed Time.vi"("Reset"=w186, "Timeout Period"="Watchdog Timeout Period (ticks)", "Current Time"=w190) -> ("Timeout"=w185:bool, "Elapsed Time"=→"Time Since Last Pet":u64)  [unwired: 7 in]
        n113 = case shown="True" w185 {
          frame False {
            # "Timeout has not expired."
          }
          frame True {
            # "#CodeRecommended - Ensure that your application behaves safely when System Reset is called. Depending on your chassis, System Reset may not keep the FPGA running or place it in the user-defined safe state. Refer to your chassis documentation to learn how System Reset behaves on your specific hardware."
            # "Timeout has expired. Reset the RT system and put the FPGA into a safe state."
            n114 = local write "Enable Watchdog"(FALSE ("Enable RT Watchdog")) -> ()
            n115 = xnode "FPGA I/O Node"("System Reset"=TRUE ("RT Reset on Watchdog Failure?")) -> ()  [unwired: 1 in, 1 out]
            "Watchdog Timed Out?" <- TRUE ("Watchdog Timed Out?")
          }
        }
      }
    }
  }
  n116 = timed-loop "Step/Direction Loop" {
    timing: w8 -> [_]
    timing-out: [_] -> w7
    stop <- FALSE stop-if-true
    n117 = global read "Global FPGA.vi" "Interpolated Position"() -> (w256:fxp<+/-,64,32>[])
    n118 = global read "Global FPGA.vi" "Reset"() -> (w250:bool[])
    n119 = global read "Global FPGA.vi" "Corrected Period"() -> (w203:u16)
    n120 = Index Array(array=w256) -> (element #1=w255:fxp<+/-,64,32>, element #2=w254:fxp<+/-,64,32>, element #3=w253:fxp<+/-,64,32>, element #4=w252:fxp<+/-,64,32>, element #5=w251:fxp<+/-,64,32>, element #6=w215:fxp<+/-,64,32>, element #7=w214:fxp<+/-,64,32>, element #8=w213:fxp<+/-,64,32>)  [unwired: 9 in, 1 out]
    n121 = Index Array(array=w250) -> (element #1=w249:bool, element #2=w248:bool, element #3=w247:bool, element #4=w246:bool, element #5=w245:bool, element #6=w212:bool, element #7=w211:bool, element #8=w210:bool)  [unwired: 9 in, 1 out]
    n122 = call "nism.step.p.fxp(modified).vi"("calls per sample"=w203, "reset"=w249, "minimum pulse"="minimum pulse", "position setpoint"=w255) -> ("steps generated"=w202:i32, "step"=w243:bool, "direction"=w244:bool)  [unwired: 4 in, 1 out]
    n123 = call "nism.step.p.fxp(modified).vi"("calls per sample"=w203, "reset"=w248, "minimum pulse"="minimum pulse", "position setpoint"=w254) -> ("steps generated"=w201:i32, "step"=w241:bool, "direction"=w242:bool)  [unwired: 4 in, 1 out]
    n124 = call "nism.step.p.fxp(modified).vi"("calls per sample"=w203, "reset"=w247, "minimum pulse"="minimum pulse", "position setpoint"=w253) -> ("steps generated"=w200:i32, "step"=w239:bool, "direction"=w240:bool)  [unwired: 4 in, 1 out]
    n125 = call "nism.step.p.fxp(modified).vi"("calls per sample"=w203, "reset"=w246, "minimum pulse"="minimum pulse", "position setpoint"=w252) -> ("steps generated"=w199:i32, "step"=w237:bool, "direction"=w238:bool)  [unwired: 4 in, 1 out]
    n126 = call "nism.step.p.fxp(modified).vi"("calls per sample"=w203, "reset"=w245, "minimum pulse"="minimum pulse", "position setpoint"=w251) -> ("steps generated"=w198:i32, "step"=w235:bool, "direction"=w236:bool)  [unwired: 4 in, 1 out]
    n127 = call "nism.step.p.fxp(modified).vi"("calls per sample"=w203, "reset"=w212, "minimum pulse"="minimum pulse", "position setpoint"=w215) -> ("steps generated"=w197:i32, "step"=w221:bool, "direction"=w222:bool)  [unwired: 4 in, 1 out]
    n128 = call "nism.step.p.fxp(modified).vi"("calls per sample"=w203, "reset"=w211, "minimum pulse"="minimum pulse", "position setpoint"=w214) -> ("steps generated"=w196:i32, "step"=w219:bool, "direction"=w220:bool)  [unwired: 4 in, 1 out]
    n129 = call "nism.step.p.fxp(modified).vi"("calls per sample"=w203, "reset"=w210, "minimum pulse"="minimum pulse", "position setpoint"=w213) -> ("steps generated"=w195:i32, "step"=w217:bool, "direction"=w218:bool)  [unwired: 4 in, 1 out]
    n130 = shared-variable "NI-sbRIO9606-018BB5CF\\User-Defined Variables\\Axis 1.Steps Generated"(w202) -> ()  [unwired: 1 in, 1 out]
    n131 = shared-variable "NI-sbRIO9606-018BB5CF\\User-Defined Variables\\Axis 2.Steps Generated"(w201) -> ()  [unwired: 1 in, 1 out]
    n132 = shared-variable "NI-sbRIO9606-018BB5CF\\User-Defined Variables\\Axis 3.Steps Generated"(w200) -> ()  [unwired: 1 in, 1 out]
    n133 = shared-variable "NI-sbRIO9606-018BB5CF\\User-Defined Variables\\Axis 4.Steps Generated"(w199) -> ()  [unwired: 1 in, 1 out]
    n134 = shared-variable "NI-sbRIO9606-018BB5CF\\User-Defined Variables\\Axis 5.Steps Generated"(w198) -> ()  [unwired: 1 in, 1 out]
    n135 = shared-variable "NI-sbRIO9606-018BB5CF\\User-Defined Variables\\Axis 6.Steps Generated"(w197) -> ()  [unwired: 1 in, 1 out]
    n136 = shared-variable "NI-sbRIO9606-018BB5CF\\User-Defined Variables\\Axis 7.Steps Generated"(w196) -> ()  [unwired: 1 in, 1 out]
    n137 = shared-variable "NI-sbRIO9606-018BB5CF\\User-Defined Variables\\Axis 8.Steps Generated"(w195) -> ()  [unwired: 1 in, 1 out]
    n138 = shared-variable "NI-sbRIO9606-018BB5CF\\User-Defined Variables\\Axis 1.Position Feedback"(w202) -> ()  [unwired: 1 in, 1 out]
    n139 = shared-variable "NI-sbRIO9606-018BB5CF\\User-Defined Variables\\Axis 2.Position Feedback"(w201) -> ()  [unwired: 1 in, 1 out]
    n140 = shared-variable "NI-sbRIO9606-018BB5CF\\User-Defined Variables\\Axis 3.Position Feedback"(w200) -> ()  [unwired: 1 in, 1 out]
    n141 = shared-variable "NI-sbRIO9606-018BB5CF\\User-Defined Variables\\Axis 4.Position Feedback"(w199) -> ()  [unwired: 1 in, 1 out]
    n142 = shared-variable "NI-sbRIO9606-018BB5CF\\User-Defined Variables\\Axis 5.Position Feedback"(w198) -> ()  [unwired: 1 in, 1 out]
    n143 = shared-variable "NI-sbRIO9606-018BB5CF\\User-Defined Variables\\Axis 6.Position Feedback"(w197) -> ()  [unwired: 1 in, 1 out]
    n144 = shared-variable "NI-sbRIO9606-018BB5CF\\User-Defined Variables\\Axis 7.Position Feedback"(w196) -> ()  [unwired: 1 in, 1 out]
    n145 = shared-variable "NI-sbRIO9606-018BB5CF\\User-Defined Variables\\Axis 8.Position Feedback"(w195) -> ()  [unwired: 1 in, 1 out]
    n146 = case shown="False" "STEP or CW? (T=STEP)" {
      tunnel: w244 -> [w290 w322]
      tunnel: w243 -> [w289 w312]
      tunnel: w242 -> [w288 w320]
      tunnel: w241 -> [w287 w310]
      tunnel: w240 -> [w286 w318]
      tunnel: w239 -> [w285 w308]
      tunnel: w238 -> [w284 w316]
      tunnel: w237 -> [w283 w306]
      tunnel: w236 -> [w282 w314]
      tunnel: w235 -> [w281 w304]
      tunnel: "Invert direction?" -> [w270 w323]
      tunnel: [w280 w321] -> w233
      tunnel: [w279 w311] -> w224
      tunnel: [w278 w319] -> w232
      tunnel: [w277 w309] -> w231
      tunnel: [w276 w317] -> w230
      tunnel: [w275 w307] -> w229
      tunnel: [w274 w315] -> w228
      tunnel: [w273 w305] -> w227
      tunnel: [w272 w313] -> w226
      tunnel: [w271 w303] -> w225
      tunnel: w222 -> [w269 w302]
      tunnel: w221 -> [w268 w301]
      tunnel: w220 -> [w267 w300]
      tunnel: w219 -> [w266 w299]
      tunnel: w218 -> [w265 w298]
      tunnel: w217 -> [w264 w297]
      tunnel: [w263 w296] -> w209
      tunnel: [w262 w295] -> w208
      tunnel: [w260 w294] -> w207
      tunnel: [w261 w293] -> w206
      tunnel: [w259 w292] -> w205
      tunnel: [w258 w291] -> w204
      frame False {
        n147 = call "Step_Dir_to_CW_CCW.vi"("invert"=w270, "step"=w289, "direction"=w290) -> ("CCW"=w279:bool, "CW"=w280:bool)  [unwired: 7 in]
        n148 = call "Step_Dir_to_CW_CCW.vi"("invert"=w270, "step"=w287, "direction"=w288) -> ("CCW"=w277:bool, "CW"=w278:bool)  [unwired: 7 in]
        n149 = call "Step_Dir_to_CW_CCW.vi"("invert"=w270, "step"=w285, "direction"=w286) -> ("CCW"=w275:bool, "CW"=w276:bool)  [unwired: 7 in]
        n150 = call "Step_Dir_to_CW_CCW.vi"("invert"=w270, "step"=w283, "direction"=w284) -> ("CCW"=w273:bool, "CW"=w274:bool)  [unwired: 7 in]
        n151 = call "Step_Dir_to_CW_CCW.vi"("invert"=w270, "step"=w281, "direction"=w282) -> ("CCW"=w271:bool, "CW"=w272:bool)  [unwired: 7 in]
        n152 = call "Step_Dir_to_CW_CCW.vi"("invert"=w270, "step"=w268, "direction"=w269) -> ("CCW"=w262:bool, "CW"=w263:bool)  [unwired: 7 in]
        n153 = call "Step_Dir_to_CW_CCW.vi"("invert"=w270, "step"=w266, "direction"=w267) -> ("CCW"=w261:bool, "CW"=w260:bool)  [unwired: 7 in]
        n154 = call "Step_Dir_to_CW_CCW.vi"("invert"=w270, "step"=w264, "direction"=w265) -> ("CCW"=w258:bool, "CW"=w259:bool)  [unwired: 7 in]
      }
      frame True {
        n155 = case shown="False" w323 {
          tunnel: w322 -> [w339 w363]
          tunnel: [w339 w362] -> w321
          tunnel: w320 -> [w337 w361]
          tunnel: [w337 w360] -> w319
          tunnel: w318 -> [w335 w359]
          tunnel: [w335 w358] -> w317
          tunnel: w316 -> [w333 w357]
          tunnel: [w333 w356] -> w315
          tunnel: w314 -> [w331 w355]
          tunnel: [w331 w354] -> w313
          tunnel: w312 -> [w338 w353]
          tunnel: [w338 w353] -> w311
          tunnel: w310 -> [w336 w352]
          tunnel: [w336 w352] -> w309
          tunnel: w308 -> [w334 w351]
          tunnel: [w334 w351] -> w307
          tunnel: w306 -> [w332 w350]
          tunnel: [w332 w350] -> w305
          tunnel: w304 -> [w330 w349]
          tunnel: [w330 w349] -> w303
          tunnel: w302 -> [w329 w348]
          tunnel: w301 -> [w328 w341]
          tunnel: w300 -> [w327 w347]
          tunnel: w299 -> [w326 w343]
          tunnel: w298 -> [w325 w346]
          tunnel: w297 -> [w324 w344]
          tunnel: [w329 w340] -> w296
          tunnel: [w328 w341] -> w295
          tunnel: [w327 w342] -> w294
          tunnel: [w326 w343] -> w293
          tunnel: [w325 w345] -> w292
          tunnel: [w324 w344] -> w291
          frame False {
          }
          frame True {
            n156 = Not(x=w347) -> (.not. x?=w342:bool)
            n157 = Not(x=w346) -> (.not. x?=w345:bool)
            n158 = Not(x=w363) -> (.not. x?=w362:bool)
            n159 = Not(x=w361) -> (.not. x?=w360:bool)
            n160 = Not(x=w359) -> (.not. x?=w358:bool)
            n161 = Not(x=w357) -> (.not. x?=w356:bool)
            n162 = Not(x=w355) -> (.not. x?=w354:bool)
            n163 = Not(x=w348) -> (.not. x?=w340:bool)
          }
        }
      }
    }
    n164 = xnode "FPGA I/O Node"("Axis1_CW"=w233, "Axis1_CCW"=w224, "Axis2_CW"=w232, "Axis2_CCW"=w231, "Axis3_CW"=w230, "Axis3_CCW"=w229, "Axis4_CW"=w228, "Axis4_CCW"=w227, "Axis5_CW"=w226, "Axis5_CCW"=w225, "RMC/DIO10"=w209, "RMC/DIO11"=w208, "RMC/DIO12"=w207, "RMC/DIO13"=w206, "RMC/DIO15"=w205, "RMC/DIO17"=w204) -> ()  [unwired: 16 in, 16 out]
  }
  n165 = timed-loop "Synchronization Loop" {
    timing: w6 -> [_]
    timing-out: [_] -> w5
    stop <- FALSE stop-if-true
    n166 = xnode "FPGA I/O Node"() -> ("Scan Clock"=w370:bool)  [unwired: 1 in, 1 out]
    n167 = global read "Global FPGA.vi" "Sync Enable"() -> (w369:bool)
    n168 = Select(t="Sync Value", s="Sync Enable override?", f=w369) -> (s? t:f=w366:bool)
    n169 = call-poly <vilib>:"nism.scan.generateSyncScan.vi"("Scan Enable?"=w366, "Scan Clock"=w370) -> ("Timer Control"=w371:T5)  [unwired: 3 in]
    n170 = global write "Global FPGA.vi" "Timer Control"(w371) -> ()
  }
  n171 = while {
    shift-right: [w377] -> _
    shift-left: FALSE ("RT Reset on Watchdog Failure?") -> [w376]
    stop <- FALSE stop-if-true
    # "Blink Loop"
    n172 = xnode "FPGA I/O Node"("FPGA LED"=w376) -> ()  [unwired: 1 in, 1 out]
    n173 = call "Wait"("Count(mSec)"=u8 100) -> ()  [unwired: 1 out]
    n174 = Not(x=w376) -> (.not. x?=w377:bool)
  }
  n175 = while "DIO Port A" {
    stop <- FALSE stop-if-true
    # "\"Reset I/O\""
    n176 = shared-variable "NI-sbRIO9606-018BB5CF\\User-Defined Variables\\Axis 1.DIO Control (Port A)"() -> (w400:u32)  [unwired: 1 in, 1 out]
    n177 = shared-variable "NI-sbRIO9606-018BB5CF\\User-Defined Variables\\Axis 2.DIO Control (Port A)"() -> (w399:u32)  [unwired: 1 in, 1 out]
    n178 = shared-variable "NI-sbRIO9606-018BB5CF\\User-Defined Variables\\Axis 3.DIO Control (Port A)"() -> (w398:u32)  [unwired: 1 in, 1 out]
    n179 = shared-variable "NI-sbRIO9606-018BB5CF\\User-Defined Variables\\Axis 4.DIO Control (Port A)"() -> (w397:u32)  [unwired: 1 in, 1 out]
    n180 = shared-variable "NI-sbRIO9606-018BB5CF\\User-Defined Variables\\Axis 5.DIO Control (Port A)"() -> (w396:u32)  [unwired: 1 in, 1 out]
    n181 = shared-variable "NI-sbRIO9606-018BB5CF\\User-Defined Variables\\Axis 6.DIO Control (Port A)"() -> (w395:u32)  [unwired: 1 in, 1 out]
    n182 = shared-variable "NI-sbRIO9606-018BB5CF\\User-Defined Variables\\Axis 7.DIO Control (Port A)"() -> (w394:u32)  [unwired: 1 in, 1 out]
    n183 = shared-variable "NI-sbRIO9606-018BB5CF\\User-Defined Variables\\Axis 8.DIO Control (Port A)"() -> (w393:u32)  [unwired: 1 in, 1 out]
    n184 = global read "Global FPGA.vi" "DIO Port A Config"() -> (w380:T10)
    n185 = Build Array(w400, w399, w398, w397, w396, w395, w394, w393) -> (w392:u32[])
    n186 = for {
      tunnel: [w419] -> w391 mode=indexing
      tunnel: w392 -> [w418] mode=indexing
      tunnel: w380 -> [w408]
      tunnel: FALSE ("Reset I/O") -> [w406]
      tunnel: T9 {"reverse limit"=FALSE, "forward limit"=FALSE, "home switch"=FALSE, "digital input 0"=FALSE, "digital input 1"=FALSE, "digital input 2"=FALSE, "digital input 3"=FALSE} ("$(driveInterface.digitalInputs.shortName)") -> [w405]
      tunnel: "Axis Digital Inputs (U8)" -> [w402] mode=indexing
      # "#note Not reading the digital outputs for now,\njust using it for the \"latch\" number"
      n187 = Unbundle By Name(w408) -> ("digital filter (us)"=w416:u16[], "safe state"=w407:enum16{"Low", "High", "No Change"}[])
      n188 = call-poly <vilib>:"nism.digitalFilter.vi"("filter value (us)"=w416, "input signal"=w402) -> ("output signal"=w404:u8)  [unwired: 9 in]
      n189 = call-poly <vilib>:"nism.interpretDIOControl.portA.2.vi"("reset"=w406, "dio control(port a)"=w418, "safe state"=w407) -> ("reset latches"=w420:u8)  [unwired: 5 in, 1 out]
      n190 = Number To Boolean Array(number=w404) -> (Boolean array=w403:bool[])
      n191 = Index Array(array=w403) -> (element #1=w415:bool, element #2=w414:bool, element #3=w413:bool, element #4=w412:bool, element #5=w411:bool, element #6=w410:bool, element #7=w409:bool)  [unwired: 7 in]
      n192 = Bundle By Name(cluster=w405, "reverse limit"=w415, "forward limit"=w414, "home switch"=w413, "digital input 0"=w412, "digital input 1"=w411, "digital input 2"=w410, "digital input 3"=w409) -> (w417:T9)
      n193 = call-poly <vilib>:"nism.generateDIOStatus.portA.vi"("digital inputs"=w417, "reset latches"=w420) -> ("dio status(port a)"=w419:u32)  [unwired: 7 in]
    }
    n194 = Index Array(array=w391) -> (element #1=w390:u32, element #2=w389:u32, element #3=w388:u32, element #4=w387:u32, element #5=w386:u32, element #6=w385:u32, element #7=w384:u32, element #8=w383:u32)  [unwired: 8 in]
    n195 = shared-variable "NI-sbRIO9606-018BB5CF\\User-Defined Variables\\Axis 1.DIO Status (Port A)"(w390) -> ()  [unwired: 1 in, 1 out]
    n196 = shared-variable "NI-sbRIO9606-018BB5CF\\User-Defined Variables\\Axis 2.DIO Status (Port A)"(w389) -> ()  [unwired: 1 in, 1 out]
    n197 = shared-variable "NI-sbRIO9606-018BB5CF\\User-Defined Variables\\Axis 3.DIO Status (Port A)"(w388) -> ()  [unwired: 1 in, 1 out]
    n198 = shared-variable "NI-sbRIO9606-018BB5CF\\User-Defined Variables\\Axis 4.DIO Status (Port A)"(w387) -> ()  [unwired: 1 in, 1 out]
    n199 = shared-variable "NI-sbRIO9606-018BB5CF\\User-Defined Variables\\Axis 5.DIO Status (Port A)"(w386) -> ()  [unwired: 1 in, 1 out]
    n200 = shared-variable "NI-sbRIO9606-018BB5CF\\User-Defined Variables\\Axis 6.DIO Status (Port A)"(w385) -> ()  [unwired: 1 in, 1 out]
    n201 = shared-variable "NI-sbRIO9606-018BB5CF\\User-Defined Variables\\Axis 7.DIO Status (Port A)"(w384) -> ()  [unwired: 1 in, 1 out]
    n202 = shared-variable "NI-sbRIO9606-018BB5CF\\User-Defined Variables\\Axis 8.DIO Status (Port A)"(w383) -> ()  [unwired: 1 in, 1 out]
  }
  n203 = timed-loop "Reset Monitoring Loop" {
    timing: w4 -> [_]
    timing-out: [_] -> w3
    stop <- FALSE stop-if-true
    n204 = global read "Global FPGA.vi" "Reset Pending"() -> (w423:bool[])
    n205 = xnode "FPGA I/O Node"() -> ("Scan Clock"=w422:bool)  [unwired: 1 in, 1 out]
    n206 = feedback-in #1(w422) -> ()
    n207 = feedback #1() -> (w421:bool)  [unwired: 1 in]
    n208 = Greater?(x=w422, y=w421) -> (0:w427:bool)
    n209 = feedback #2() -> (w426:bool[])  [unwired: 1 in]
    n210 = Select(t=w423, s=w427, f=w426) -> (s? t:f=w424:bool[])
    n211 = feedback-in #2(w424) -> ()
    n212 = global write "Global FPGA.vi" "Reset"(w424) -> ()
  }
  n213 = node-c288(w3) -> ()
  n214 = node-c288(w5) -> ()
  n215 = node-c288(w7) -> ()
